vi "Partition(String).vi"(8 "Indices In":i32[](array[numeric]), 9 "hi":i32, 10 "lo":i32, 11 "Array In":string[](array[string])) -> (0 "Indices Out":i32[](array[numeric]), 2 "pivot":i32, 3 "Array Out":string[](array[string]))   [LabVIEW 2015, in "Sorting.lvlib"]
uses:
  Sorting.lvlib
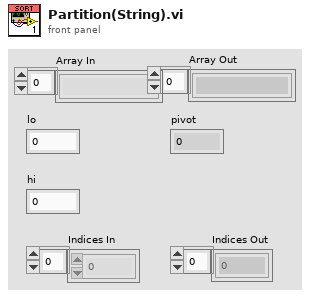
[diagram p1: front panel]
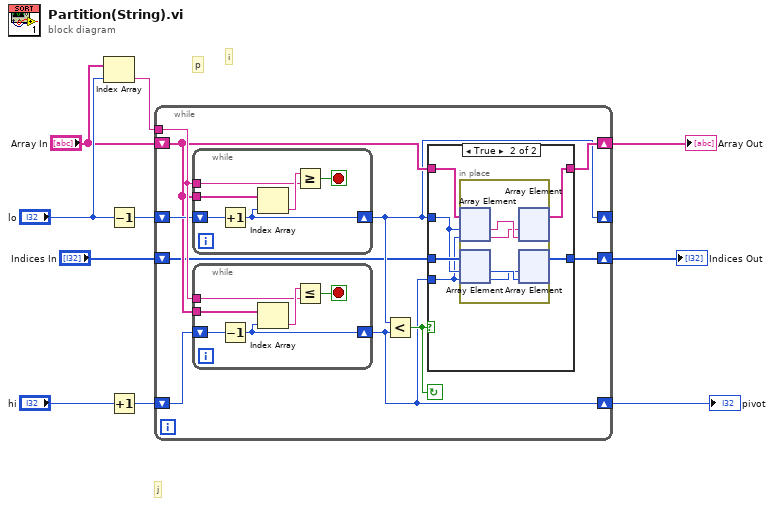
[diagram p0: block diagram]
diagram:
  # "p"
  # "j"
  # "i"
  n1 = Index Array(array="Array In", index="lo") -> (element=w6:string)
  n2 = Decrement(x="lo") -> (x-1=w5:i32)
  n3 = Increment(x="hi") -> (x+1=w8:i32)
  n4 = while {
    tunnel: w6 -> [w20]
    shift-right: [w17] -> w3
    shift-left: "Array In" -> [w18]
    shift-right: [w13] -> _
    shift-left: w5 -> [w19]
    shift-right: [w14] -> w4
    shift-left: w8 -> [w15]
    shift-right: [w11] -> w1
    shift-left: "Indices In" -> [w12]
    stop <- w16 continue-if-true
    n5 = while {
      tunnel: w20 -> [w37]
      tunnel: w18 -> [w35]
      shift-right: [w33] -> w13
      shift-left: w19 -> [w34]
      stop <- w36 stop-if-true
      n6 = Increment(x=w34) -> (x+1=w33:i32)
      n7 = Index Array(array=w35, index=w33) -> (element=w38:string)
      n8 = Greater Or Equal?(x=w38, y=w37) -> (x >= y?=w36:bool)
    }
    n9 = while {
      tunnel: w18 -> [w44]
      tunnel: w20 -> [w42]
      shift-right: [w39] -> w14
      shift-left: w15 -> [w40]
      stop <- w41 stop-if-true
      n10 = Decrement(x=w40) -> (x-1=w39:i32)
      n11 = Index Array(array=w44, index=w39) -> (element=w43:string)
      n12 = Less Or Equal?(x=w43, y=w42) -> (x <= y?=w41:bool)
    }
    n13 = Less?(x=w13, y=w14) -> (x < y?=w16:bool)
    n14 = case shown="True" w16 {
      tunnel: w18 -> [w22 w28]
      tunnel: w13 -> [_ w24]
      tunnel: w14 -> [_ w23]
      tunnel: [w22 w27] -> w17
      tunnel: w12 -> [w21 w26]
      tunnel: [w21 w25] -> w11
      frame False {
      }
      frame True {
        n15 = in-place {
          n16 = in-place-array #1(w28, w24, w23) -> (w32:string, w31:string)
          n17 = in-place-array #2(w26, w24, w23) -> (w30:i32, w29:i32)
          n18 = in-place-array #1(w31, w32) -> (w27:string[])  [unwired: 2 out]
          n19 = in-place-array #2(w29, w30) -> (w25:i32[])  [unwired: 2 out]
        }
      }
    }
  }
  "pivot" <- w4
  "Array Out" <- w3
  "Indices Out" <- w1
